vi "Help Window.vi"() -> ()   [LabVIEW 2017]
doc: "Displays help information and waits until Close button clicked."
panel:
  in  "close":bool
  # "Switch   Arg          Default      : Description\t\n-?                                     : Display help window\n-n        text           VI name       : Set icon main text\n-h        text           empty         : Set icon header text (do not work with -f none)\n-c        [b]|[blue]     black         : Set icon background color\n          [bl]|[black]                 :\n          [br]|[brown]                 :\n          [cr]|[cream]|[creamy]        :\n          [db]|[dark blue]             :\n          [g]|[green]                  :\n          [gr]|[gray]                  :\n          [pi]|[r]|[pink]|[red]        :\n          [vi]|[violet]                :\n          [white]                      :\n          [ye]|[yellow]                :\n-f        [none]         compact lib   : Set VI frame\n          [compact lib]                :\n-t        [none]         none          : Set text format\n------------------------------------------------------------------------------------------"
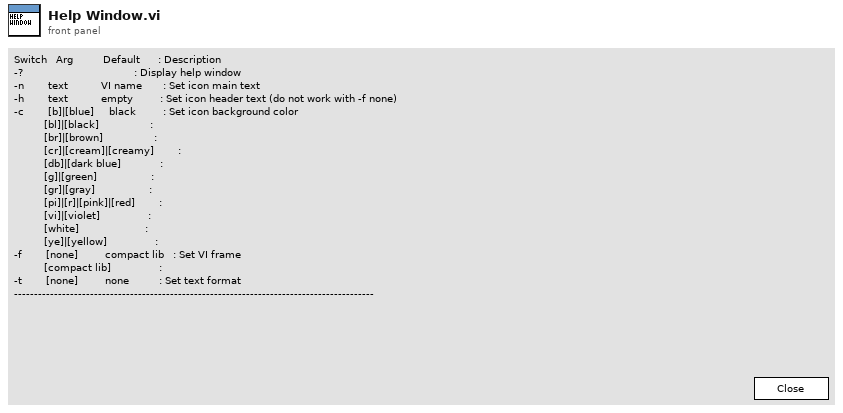
[diagram p1: front panel]
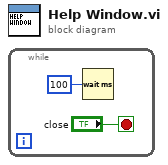
[diagram p0: block diagram]
diagram:
  n1 = while {
    stop <- "close" stop-if-true
    n2 = Wait (ms)(milliseconds to wait=u32 100) -> ()  [unwired: 1 out]
  }
